vi "sppf single step.vi"(7 "dt":dbl, 8 "num green photons":dbl, 9 "num red photons":dbl, 10 "w":dbl[][](array[numeric])=[[1000000000.0, 0.0], [0.0, 100000000.0]], 11 "theta":dbl[](array[numeric])=[0.0, 0.0]) -> (1 "wjjm1":dbl[][](array[numeric]), 2 "w":dbl[][](array[numeric]), 3 "theta":dbl[](array[numeric]))   [LabVIEW 2010]
uses:
  <vilib>/Analysis/Matrix/Datatypes/RealMatrix.ctl
  <vilib>/Analysis/baseanly.llb/Matrix Type of Inverse Matrix.ctl
  <vilib>/Analysis/Matrix/Numeric/Multiply/Multiply - R,RM.vi
  <vilib>/Analysis/Matrix/Numeric/Add/Add - RM,RM.vi
  <vilib>/Analysis/baseanly.llb/Real Inverse Matrix.vi
  <vilib>/Analysis/BLAS.llb/dgemv - General Matrix-Vector Product (DBL).vi
  <vilib>/Analysis/Matrix/NI_Matrix.lvlib
  <vilib>/Analysis/NI_AALBase.lvlib
  <vilib>/Analysis/NI_AALBLAS.lvlib
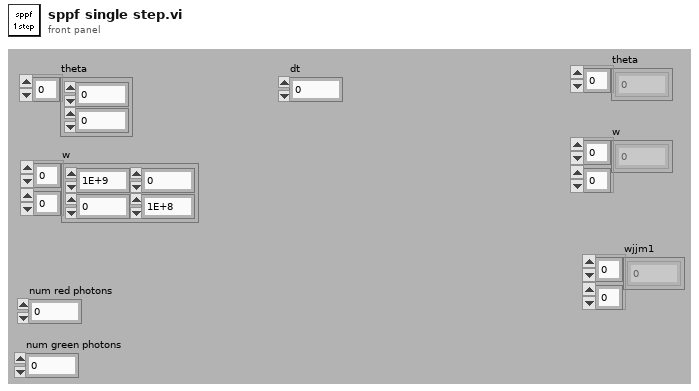
[diagram p1: front panel]
types:
  T1 = typedef "NI_AALBase.lvlib/Matrix Type of Inverse Matrix.ctl" = enum32{"General", "Positive Definite", "Lower Triangular", "Upper Triangular"}
  T2 = typedef "NI_Matrix.lvlib/RealMatrix.ctl" = dbl[][]
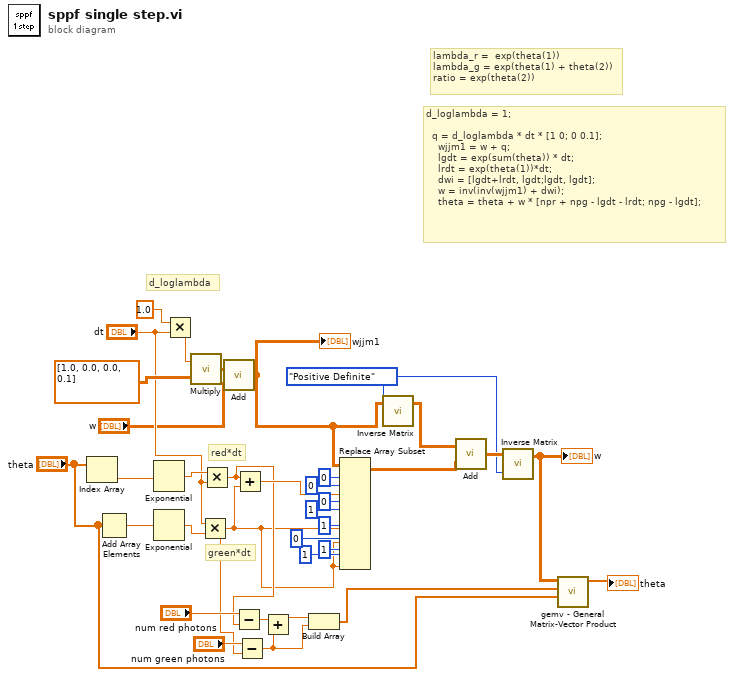
[diagram p0: block diagram]
diagram:
  w16 = Matrix_Type_of_Inverse_Matrix."Positive Definite" ("matrix type")
  # "d_loglambda = 1;\n  \n  q = d_loglambda * dt * [1 0; 0 0.1];\n    wjjm1 = w + q;\n    lgdt = exp(sum(theta)) * dt;\n    lrdt = exp(theta(1))*dt;\n    dwi = [lgdt+lrdt, lgdt;lgdt, lgdt];\n    w = inv(inv(wjjm1) + dwi);\n    theta = theta + w * [npr + npg - lgdt - lrdt; npg - lgdt];"
  # "d_loglambda"
  # "green*dt"
  # "red*dt"
  # "lambda_r =  exp(theta(1))\nlambda_g = exp(theta(1) + theta(2))\nratio = exp(theta(2))"
  n1 = Index Array(array="theta") -> (element=w33:dbl)  [unwired: 1 in]
  n2 = Add Array Elements(numeric array="theta") -> (sum=w32:dbl)
  n3 = Exponential(1:w33) -> (0:w31:dbl)
  n4 = Exponential(1:w32) -> (0:w30:dbl)
  n5 = Multiply(x=1.0, y="dt") -> (x*y=w3:dbl)
  n6 = call-poly <vilib>:"Multiply.vi"("Real Matrix A"=T2 [[1.0, 0.0], [0.0, 0.1]] ("Real Matrix"), "Real Scalar c"=w3) -> ("c * A"=w34:T2)
  n7 = Multiply(x="dt", y=w30) -> (x*y=w12:dbl)
  n8 = Multiply(x=w31, y="dt") -> (x*y=w14:dbl)
  n9 = call-poly <vilib>:"Add.vi"("Real Matrix B"="w", "Real Matrix A"=w34) -> ("A + B"=w1:T2)
  "wjjm1" <- w1
  n10 = Subtract(x="num red photons", y=w14) -> (x-y=w11:dbl)
  n11 = Add(x=w14, y=w12) -> (x+y=w20:dbl)
  n12 = Subtract(x="num green photons", y=w12) -> (x-y=w9:dbl)
  n13 = Add(x=w11, y=w9) -> (x+y=w10:dbl)
  n14 = Build Array(w10, w9) -> (w8:dbl[])
  n15 = Replace Array Subset(array=w1, new element #1=w20, index (row) #1=0 ("disabled index (row)"), index (col) #1=0 ("disabled index (col)"), new element #2=w12, index (row) #2=0 ("index (row)"), index (col) #2=1 ("disabled index (col)"), new element #3=w12, index (row) #3=1 ("index (row)"), index (col) #3=0 ("disabled index (col)"), new element #4=w12, index (row) #4=1 ("index (row)"), index (col) #4=1 ("disabled index (col)")) -> (w18:T2)
  n16 = call-poly <vilib>:"Inverse Matrix.vi"("matrix type"=w16, "Input Matrix"=w1) -> ("Inverse Matrix"=w19:T2)  [unwired: 1 out]
  n17 = call-poly <vilib>:"Add.vi"("Real Matrix B"=w18, "Real Matrix A"=w19) -> ("A + B"=w17:T2)
  n18 = call-poly <vilib>:"Inverse Matrix.vi"("matrix type"=w16, "Input Matrix"=w17) -> ("Inverse Matrix"=w6:T2)  [unwired: 1 out]
  "w" <- w6
  n19 = call-poly <vilib>:"gemv - General Matrix-Vector Product.vi"("y"="theta", "x"=w8, "A"=w6) -> ("dgemv"=→"theta":dbl[])  [unwired: 7 in, 1 out]
